vi "Write Name.vi"(8 "error in (no error)":errorcluster, 10 "Name":string, 11 "BaseResponder in":refnum<class "BaseResponder.lvclass">) -> (0 "error out":errorcluster, 3 "BaseResponder out":refnum<class "BaseResponder.lvclass">)   [LabVIEW 2013, in "BaseResponder.lvclass"]
doc: "The Name of the responder is part of each response it sends and is used to identify the owning driver"
uses:
  BaseResponder.lvclass
  BaseResponder.lvclass/BaseResponder.ctl
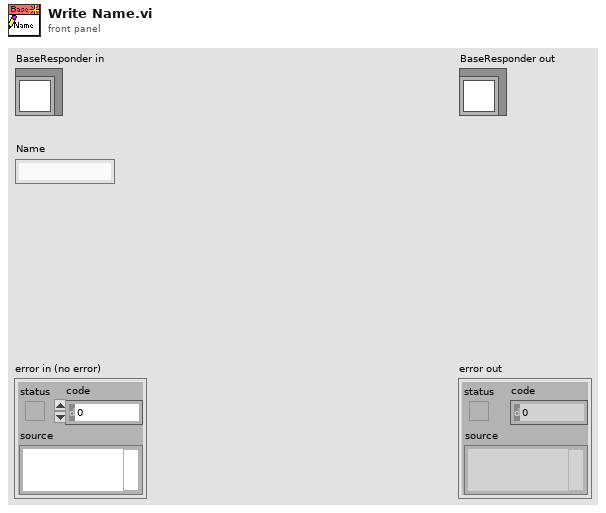
[diagram p1: front panel]
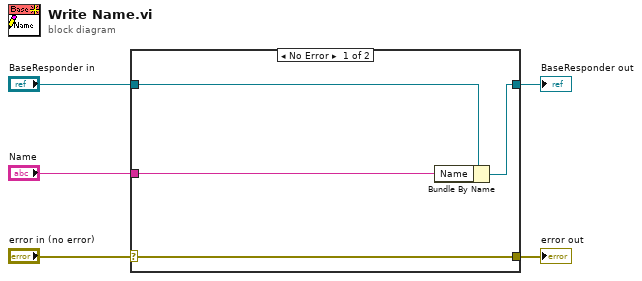
[diagram p0: block diagram]
diagram:
  n1 = case shown="No Error" "error in (no error)" {
    selector: "error in (no error)" -> [w9 w10]
    tunnel: [w9 w10] -> w4
    tunnel: [w7 w11] -> w2
    tunnel: "BaseResponder in" -> [w8 w11]
    tunnel: "Name" -> [w6 _]
    frame No Error {
      n2 = Bundle By Name(cluster=w8, "Name"=w6) -> (w7:refnum<class "BaseResponder.lvclass">)
    }
    frame Error {
    }
  }
  "error out" <- w4
  "BaseResponder out" <- w2
